vi "RealTime_MatLab_Simulink.vi"() -> ()   [LabVIEW 2024]
uses:
  <vilib>/Utility/error.llb/Trim Whitespace One-Sided.vi
panel:
  in  "Tab Control":enum32{""}(tab)
  out "Alarm RS":bool
  out "Alarm PM":bool
  out "Alarm VC":bool
  out "Alarm VB":bool
  out "Alarm VA":bool
  out "Alarm CB":bool
  out "Alarm CC":bool
  out "Alarm CA":bool
  out "Voltage B":bool
  out "Rotor speed (pu)":dbl format="%#_10f"
  out "Mechanical power (pu)":dbl format="%#_10f"
  out "Voltage C (pu)":dbl format="%#_10f"
  out "Voltage B (pu)":dbl format="%#_10f"
  out "Rotor speed (pu)":dbl(graph)
  out "Mechanical power (pu)":dbl(graph)
  out "Voltage C (pu)":dbl(graph)
  out "Voltage B":dbl(graph)
  out "Rotor speed":bool
  out "Pm":bool
  out "Voltage C":bool
  out "Current B":bool
  out "Current C":bool
  out "Volatge A":bool
  out "Current A":bool
  out "Voltage A (pu)":dbl format="%#_10f"
  out "Current C (pu)":dbl format="%#_10f"
  out "Current B (pu)":dbl format="%#_10f"
  out "Current A (pu)":dbl format="%#_10f"
  out "Voltage A (pu)":dbl(graph)
  out "Current C (pu)":dbl(graph)
  out "Current B (pu)":dbl(graph)
  out "Current A (pu)":dbl(graph)
  # "HUMAN MACHINE INTERFACE: CONTROL PANEL - REALTIME SUPERVISION INTERFACE  MATLAB/SIMULINK HYDROPOWER"
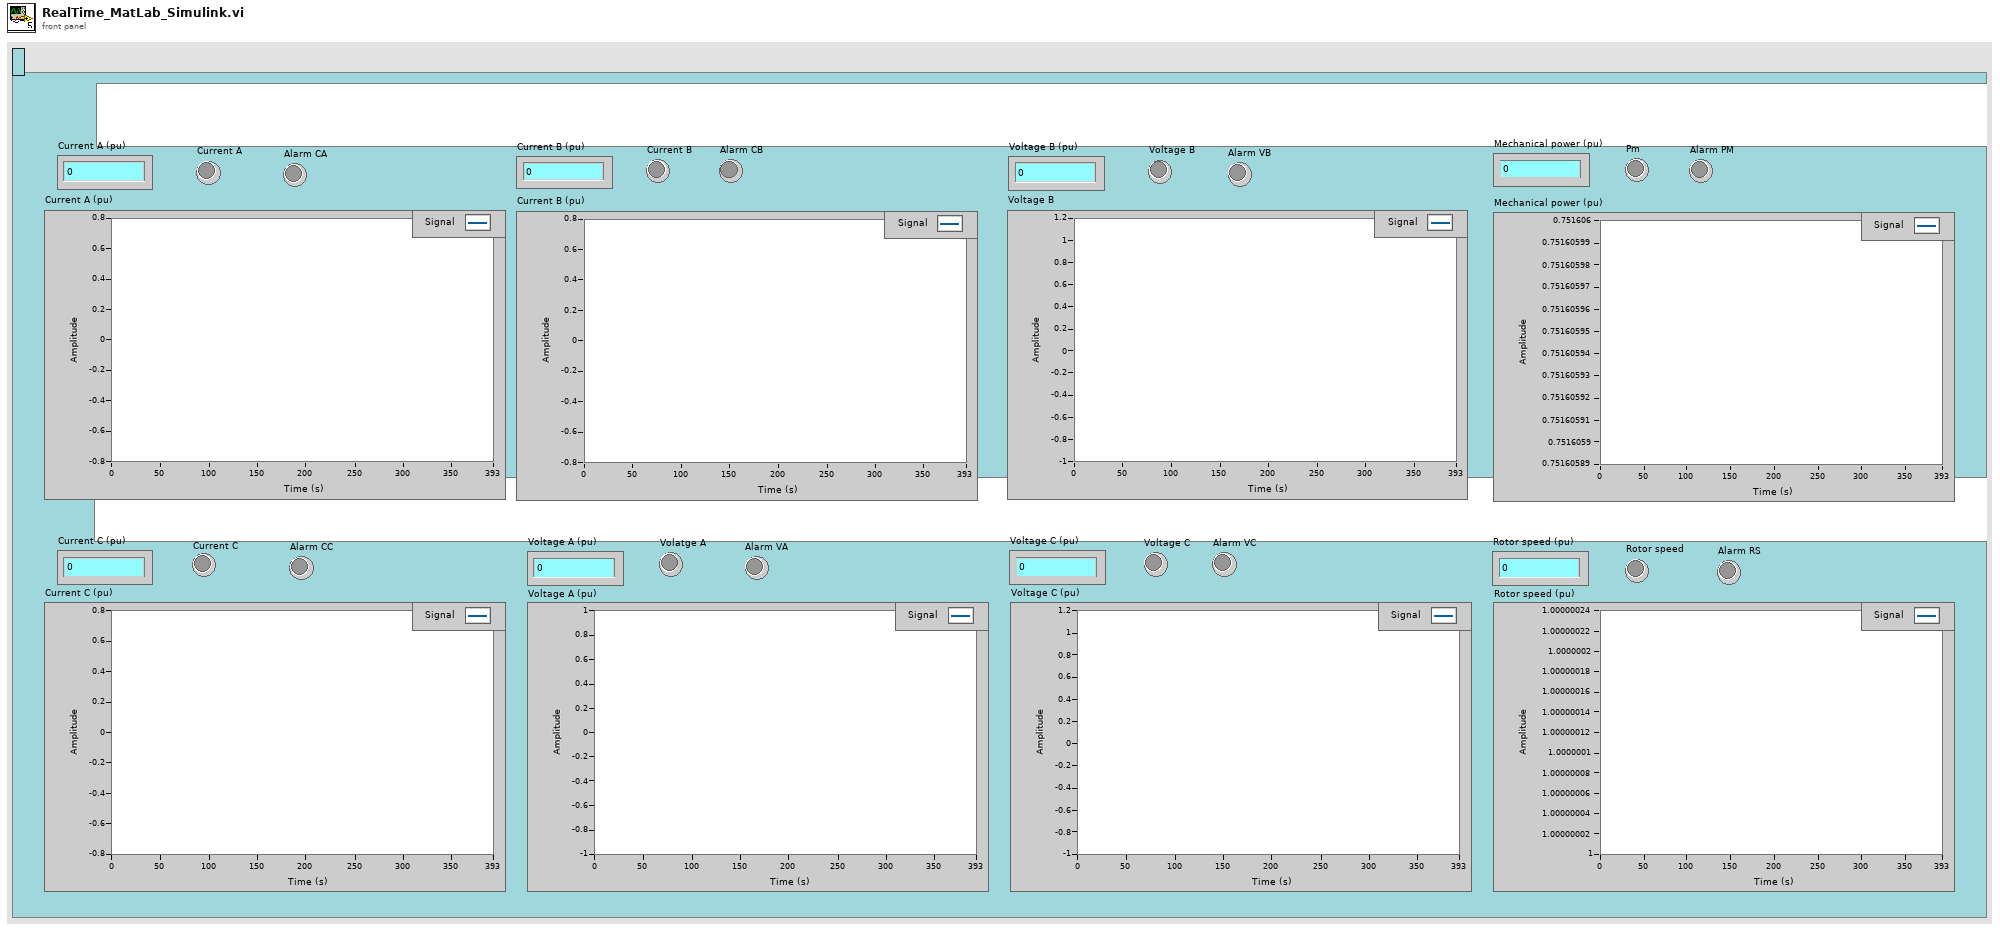
[diagram p1: front panel]
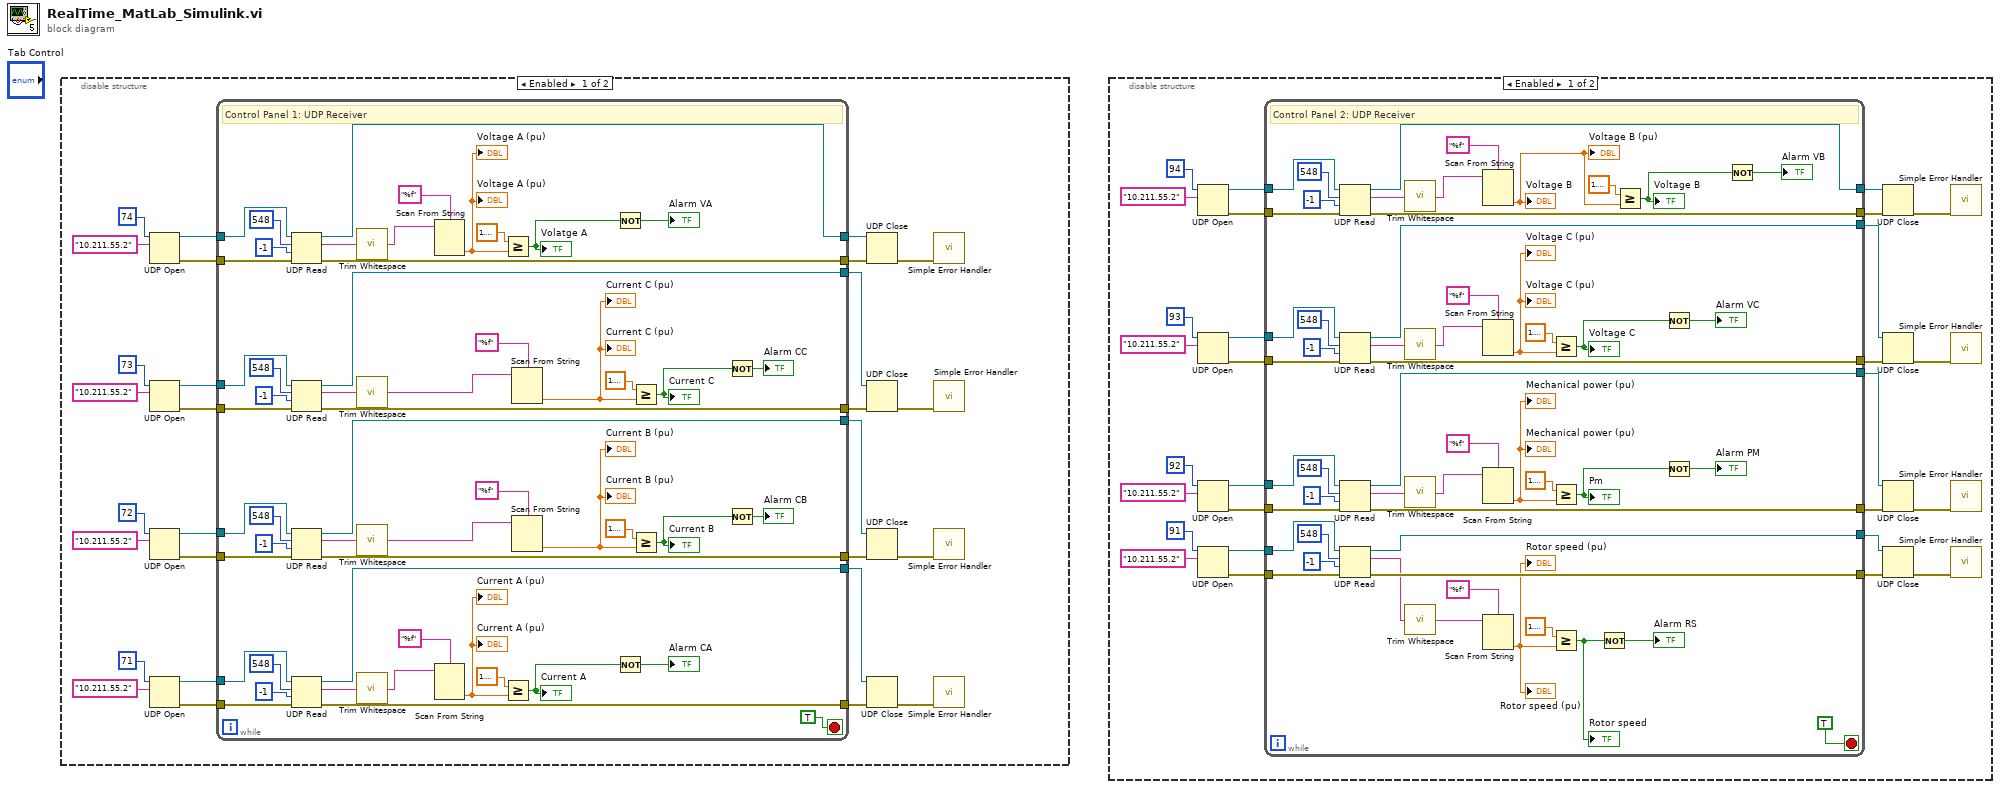
[diagram p0: block diagram]
diagram:
  n1 = disable-structure shown="Enabled" {
    frame Enabled {
      n2 = UDP Open(10:"10.211.55.2" ("service name"), 11:u16 74 ("port")) -> (port=w8:refnum<k16>, 0:w6:errorcluster)  [unwired: 3 in, 1 out]
      n3 = UDP Open(10:"10.211.55.2" ("service name"), 11:u16 73 ("port")) -> (port=w14:refnum<k16>, 0:w12:errorcluster)  [unwired: 3 in, 1 out]
      n4 = UDP Open(10:"10.211.55.2" ("service name"), 11:u16 72 ("port")) -> (port=w20:refnum<k16>, 0:w22:errorcluster)  [unwired: 3 in, 1 out]
      n5 = UDP Open(10:"10.211.55.2" ("service name"), 11:u16 71 ("port")) -> (port=w26:refnum<k16>, 0:w25:errorcluster)  [unwired: 3 in, 1 out]
      n6 = while {
        tunnel: w26 -> [w81]
        tunnel: w25 -> [w80]
        tunnel: [w79] -> w24
        tunnel: [w78] -> w23
        tunnel: w22 -> [w77]
        tunnel: [w74] -> w21
        tunnel: w20 -> [w76]
        tunnel: [w75] -> w19
        tunnel: w14 -> [w73]
        tunnel: [w72] -> w13
        tunnel: w12 -> [w71]
        tunnel: [w70] -> w11
        tunnel: w8 -> [w69]
        tunnel: [w68] -> w7
        tunnel: w6 -> [w67]
        tunnel: [w66] -> w5
        stop <- TRUE stop-if-true
        # "Control Panel 1: UDP Receiver"
        n7 = UDP Read(connection ID=w69, max size (548)=548, timeout ms (25000)=-1, 8:w67) -> (data out=w53:string, error out=w66:errorcluster, 3:w68:refnum<k16>)  [unwired: 2 out]
        n8 = UDP Read(connection ID=w73, max size (548)=548, timeout ms (25000)=-1, 8:w71) -> (data out=w54:string, error out=w70:errorcluster, 3:w72:refnum<k16>)  [unwired: 2 out]
        n9 = UDP Read(connection ID=w76, max size (548)=548, timeout ms (25000)=-1, 8:w77) -> (data out=w55:string, error out=w74:errorcluster, 3:w75:refnum<k16>)  [unwired: 2 out]
        n10 = UDP Read(connection ID=w81, max size (548)=548, timeout ms (25000)=-1, 8:w80) -> (data out=w56:string, error out=w79:errorcluster, 3:w78:refnum<k16>)  [unwired: 2 out]
        n11 = call <vilib>:"Trim Whitespace.vi"("string"=w53) -> ("trimmed string"=w52:string)  [unwired: 1 in]
        n12 = call <vilib>:"Trim Whitespace.vi"("string"=w54) -> ("trimmed string"=w50:string)  [unwired: 1 in]
        n13 = call <vilib>:"Trim Whitespace.vi"("string"=w55) -> ("trimmed string"=w48:string)  [unwired: 1 in]
        n14 = call <vilib>:"Trim Whitespace.vi"("string"=w56) -> ("trimmed string"=w46:string)  [unwired: 1 in]
        n15 = Scan From String(format string="%f", input string=w52) -> (output 1=w51:dbl)  [unwired: 3 in, 3 out]
        "Voltage A (pu)" <- w51
        "Voltage A (pu)" <- w51
        n16 = Scan From String(format string="%f", input string=w46) -> (output 1=w45:dbl)  [unwired: 3 in, 3 out]
        "Current A (pu)" <- w45
        "Current A (pu)" <- w45
        n17 = Greater Or Equal?(x=1.5000000000000002, y=w51) -> (x >= y?=w34:bool)
        "Volatge A" <- w34
        n18 = Greater Or Equal?(x=1.5000000000000002, y=w45) -> (x >= y?=w31:bool)
        "Current A" <- w31
        n19 = Scan From String(format string="%f", input string=w50) -> (output 1=w49:dbl)  [unwired: 3 in, 3 out]
        "Current C (pu)" <- w49
        "Current C (pu)" <- w49
        n20 = Scan From String(format string="%f", input string=w48) -> (output 1=w47:dbl)  [unwired: 3 in, 3 out]
        "Current B (pu)" <- w47
        "Current B (pu)" <- w47
        n21 = Not(x=w34) -> (.not. x?=→"Alarm VA":bool)
        n22 = Not(x=w31) -> (.not. x?=→"Alarm CA":bool)
        n23 = Greater Or Equal?(x=1.5000000000000002, y=w49) -> (x >= y?=w37:bool)
        "Current C" <- w37
        n24 = Greater Or Equal?(x=1.5000000000000002, y=w47) -> (x >= y?=w39:bool)
        "Current B" <- w39
        n25 = Not(x=w37) -> (.not. x?=→"Alarm CC":bool)
        n26 = Not(x=w39) -> (.not. x?=→"Alarm CB":bool)
      }
      n27 = UDP Close(connection ID=w7, 8:w5) -> (error out=w1:errorcluster)  [unwired: 1 out]
      n28 = UDP Close(connection ID=w13, 8:w11) -> (error out=w2:errorcluster)  [unwired: 1 out]
      n29 = UDP Close(connection ID=w19, 8:w21) -> (error out=w3:errorcluster)  [unwired: 1 out]
      n30 = UDP Close(connection ID=w23, 8:w24) -> (error out=w4:errorcluster)  [unwired: 1 out]
      n31 = call <vilib>:"Simple Error Handler.vi"("error in (no error)"=w1) -> ()  [unwired: 4 in, 5 out]
      n32 = call <vilib>:"Simple Error Handler.vi"("error in (no error)"=w2) -> ()  [unwired: 4 in, 5 out]
      n33 = call <vilib>:"Simple Error Handler.vi"("error in (no error)"=w3) -> ()  [unwired: 4 in, 5 out]
      n34 = call <vilib>:"Simple Error Handler.vi"("error in (no error)"=w4) -> ()  [unwired: 4 in, 5 out]
    }
    frame Disabled {
    }
  }
  n35 = disable-structure shown="Enabled" {
    frame Enabled {
      n36 = UDP Open(10:"10.211.55.2" ("service name"), 11:u16 94 ("port")) -> (port=w87:refnum<k16>, 0:w89:errorcluster)  [unwired: 3 in, 1 out]
      n37 = UDP Open(10:"10.211.55.2" ("service name"), 11:u16 93 ("port")) -> (port=w95:refnum<k16>, 0:w94:errorcluster)  [unwired: 3 in, 1 out]
      n38 = UDP Open(10:"10.211.55.2" ("service name"), 11:u16 92 ("port")) -> (port=w101:refnum<k16>, 0:w100:errorcluster)  [unwired: 3 in, 1 out]
      n39 = UDP Open(10:"10.211.55.2" ("service name"), 11:u16 91 ("port")) -> (port=w107:refnum<k16>, 0:w105:errorcluster)  [unwired: 3 in, 1 out]
      n40 = while {
        tunnel: w107 -> [w162]
        tunnel: [w161] -> w106
        tunnel: w105 -> [w160]
        tunnel: [w159] -> w104
        tunnel: w101 -> [w158]
        tunnel: w100 -> [w157]
        tunnel: [w156] -> w99
        tunnel: [w155] -> w98
        tunnel: w95 -> [w154]
        tunnel: w94 -> [w153]
        tunnel: [w152] -> w93
        tunnel: [w151] -> w92
        tunnel: w89 -> [w150]
        tunnel: [w149] -> w88
        tunnel: w87 -> [w148]
        tunnel: [w147] -> w86
        stop <- TRUE stop-if-true
        # "Control Panel 2: UDP Receiver"
        n41 = UDP Read(connection ID=w148, max size (548)=548, timeout ms (25000)=-1, 8:w150) -> (data out=w134:string, error out=w149:errorcluster, 3:w147:refnum<k16>)  [unwired: 2 out]
        n42 = UDP Read(connection ID=w154, max size (548)=548, timeout ms (25000)=-1, 8:w153) -> (data out=w135:string, error out=w151:errorcluster, 3:w152:refnum<k16>)  [unwired: 2 out]
        n43 = UDP Read(connection ID=w158, max size (548)=548, timeout ms (25000)=-1, 8:w157) -> (data out=w136:string, error out=w156:errorcluster, 3:w155:refnum<k16>)  [unwired: 2 out]
        n44 = UDP Read(connection ID=w162, max size (548)=548, timeout ms (25000)=-1, 8:w160) -> (data out=w137:string, error out=w159:errorcluster, 3:w161:refnum<k16>)  [unwired: 2 out]
        n45 = call <vilib>:"Trim Whitespace.vi"("string"=w134) -> ("trimmed string"=w133:string)  [unwired: 1 in]
        n46 = call <vilib>:"Trim Whitespace.vi"("string"=w135) -> ("trimmed string"=w132:string)  [unwired: 1 in]
        n47 = call <vilib>:"Trim Whitespace.vi"("string"=w136) -> ("trimmed string"=w131:string)  [unwired: 1 in]
        n48 = call <vilib>:"Trim Whitespace.vi"("string"=w137) -> ("trimmed string"=w127:string)  [unwired: 1 in]
        n49 = Scan From String(format string="%f", input string=w133) -> (output 1=w128:dbl)  [unwired: 3 in, 3 out]
        "Voltage B" <- w128
        "Voltage B (pu)" <- w128
        n50 = Scan From String(format string="%f", input string=w132) -> (output 1=w129:dbl)  [unwired: 3 in, 3 out]
        "Voltage C (pu)" <- w129
        "Voltage C (pu)" <- w129
        n51 = Scan From String(format string="%f", input string=w131) -> (output 1=w130:dbl)  [unwired: 3 in, 3 out]
        "Mechanical power (pu)" <- w130
        "Mechanical power (pu)" <- w130
        n52 = Scan From String(format string="%f", input string=w127) -> (output 1=w126:dbl)  [unwired: 3 in, 3 out]
        "Rotor speed (pu)" <- w126
        "Rotor speed (pu)" <- w126
        n53 = Greater Or Equal?(x=1.5000000000000002, y=w129) -> (x >= y?=w114:bool)
        "Voltage C" <- w114
        n54 = Greater Or Equal?(x=1.5000000000000002, y=w130) -> (x >= y?=w117:bool)
        "Pm" <- w117
        n55 = Greater Or Equal?(x=1.5000000000000002, y=w126) -> (x >= y?=w120:bool)
        "Rotor speed" <- w120
        n56 = Not(x=w120) -> (.not. x?=→"Alarm RS":bool)
        n57 = Greater Or Equal?(x=1.5000000000000002, y=w128) -> (x >= y?=w111:bool)
        "Voltage B" <- w111
        n58 = Not(x=w114) -> (.not. x?=→"Alarm VC":bool)
        n59 = Not(x=w117) -> (.not. x?=→"Alarm PM":bool)
        n60 = Not(x=w111) -> (.not. x?=→"Alarm VB":bool)
      }
      n61 = UDP Close(connection ID=w86, 8:w88) -> (error out=w85:errorcluster)  [unwired: 1 out]
      n62 = UDP Close(connection ID=w93, 8:w92) -> (error out=w84:errorcluster)  [unwired: 1 out]
      n63 = UDP Close(connection ID=w98, 8:w99) -> (error out=w83:errorcluster)  [unwired: 1 out]
      n64 = UDP Close(connection ID=w106, 8:w104) -> (error out=w82:errorcluster)  [unwired: 1 out]
      n65 = call <vilib>:"Simple Error Handler.vi"("error in (no error)"=w85) -> ()  [unwired: 4 in, 5 out]
      n66 = call <vilib>:"Simple Error Handler.vi"("error in (no error)"=w84) -> ()  [unwired: 4 in, 5 out]
      n67 = call <vilib>:"Simple Error Handler.vi"("error in (no error)"=w83) -> ()  [unwired: 4 in, 5 out]
      n68 = call <vilib>:"Simple Error Handler.vi"("error in (no error)"=w82) -> ()  [unwired: 4 in, 5 out]
    }
    frame Disabled {
    }
  }
